vi "Read Path.vi"(8 "error in (no error)":errorcluster, 11 "Application in":refnum<class "Application.lvclass">) -> (0 "error out":errorcluster, 2 "Path":path, 3 "Application out":refnum<class "Application.lvclass">)   [LabVIEW 2015, in "Application.lvclass"]
uses:
  Application.lvclass
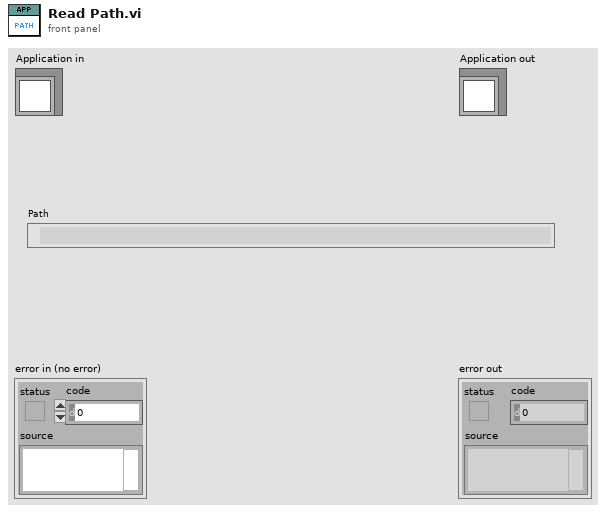
[diagram p1: front panel]
types:
  T1 = enum32{"invalid app kind", "Development System", "Run Time System", "Student Edition", "Embedded LabVIEW", "Evaluation", "Custom"}
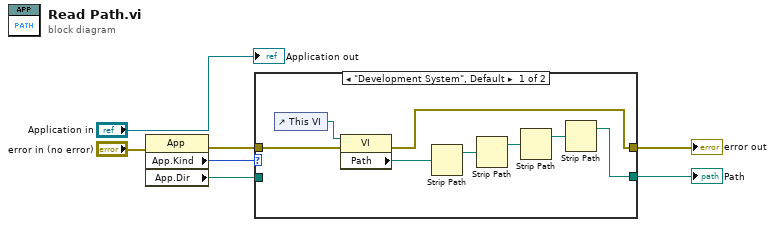
[diagram p0: block diagram]
diagram:
  n1 = property class="App"(error in="error in (no error)") -> (error out=w2:errorcluster, "App.Kind"=w6:T1, "App.Dir"=w5:path)  [unwired: 1 in, 1 out]
  n2 = case shown="\"Development System\", Default" w6 {
    tunnel: w5 -> [_ w17]
    tunnel: [w10 w17] -> w4
    tunnel: w2 -> [w9 w16]
    tunnel: [w8 w16] -> w1
    frame "Development System", Default {
      n3 = control-ref of="This VI"() -> (w15:refnum<vi>)
      n4 = property class="VI"(reference=w15, error in=w9) -> (error out=w8:errorcluster, "Path"=w14:path)  [unwired: 1 out]
      n5 = Strip Path(path=w14) -> (stripped path=w13:path)  [unwired: 1 out]
      n6 = Strip Path(path=w13) -> (stripped path=w12:path)  [unwired: 1 out]
      n7 = Strip Path(path=w12) -> (stripped path=w11:path)  [unwired: 1 out]
      n8 = Strip Path(path=w11) -> (stripped path=w10:path)  [unwired: 1 out]
    }
    frame "Run Time System" {
    }
  }
  "error out" <- w1
  "Path" <- w4
  "Application out" <- "Application in"
